vi "MGCC_FntStaMach_main_HTB.vi"() -> ()   [LabVIEW 2016]
doc: "-----------------------------------------------------------------------------------------------------------------------\nCopyright <2019> <The University of Tennessee at Knoxville and the University of Tennessee Research Foundation>\nThis software is released under BSD-3 \nhttps://opensource.org/licenses/BSD-3-Clause \nAdditional license options available at https://utrf.tennessee.edu/industry/sample-agreements/\n-----------------------------------------------------------------------------------------------------------------------\n\n\nMain function for FSM in MGCC. The inputs are flags feedback from other functions and MGLCs. The outputs are the next states and updates in sensoring datas."
panel:
  in  "i_MGCC_StaEst_breakpoint":i32=11
  in  "b_MGCC_StaEst_enable_noise":bool
  in  "b_MGCC_FntStaMach_All_Loop_Stop":bool
  out "Functions":bool[](array[boolean])
  out "Current state":string
  out "Current Time":string
  in  "Manual turn off":bool
  in  "Event manual panel":bool
  out "Bool of state":bool[](array[boolean])
  # "Finte State Machine"
  # "Energy management"
  # "State Esimation"
  # "Model Management"
  # "Data Logging"
  # "Communication"
  # "PV Forecasting"
  # "PQ Balance"
  # "Load Forecasting"
  # "BKS"
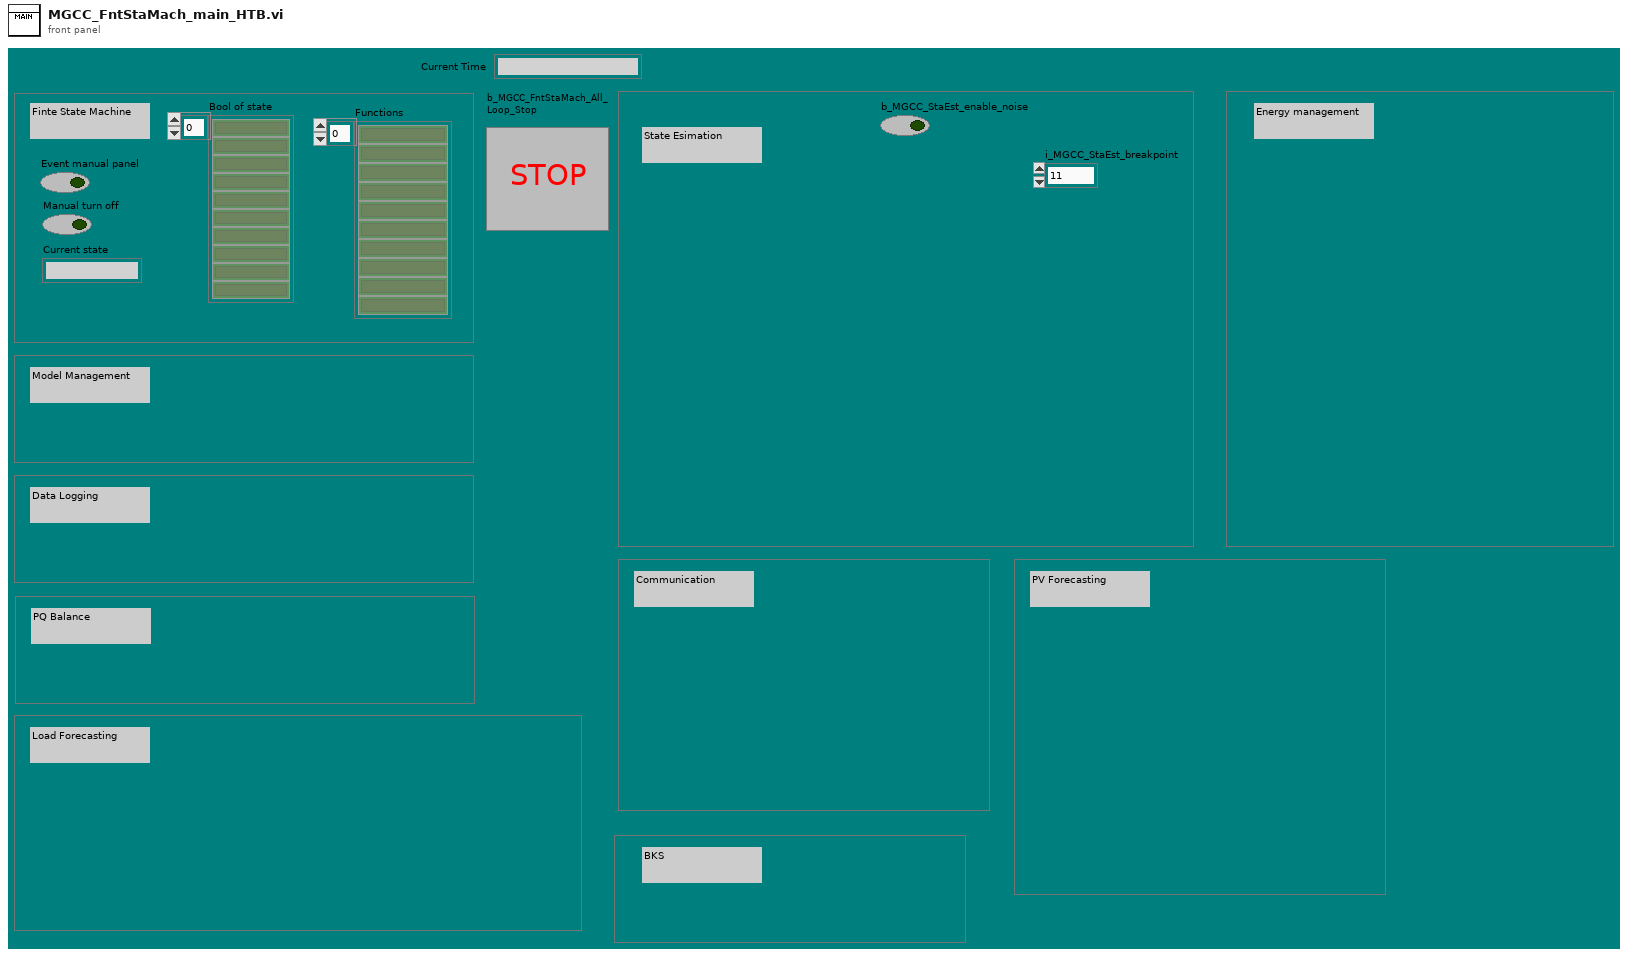
[diagram p1: front panel]
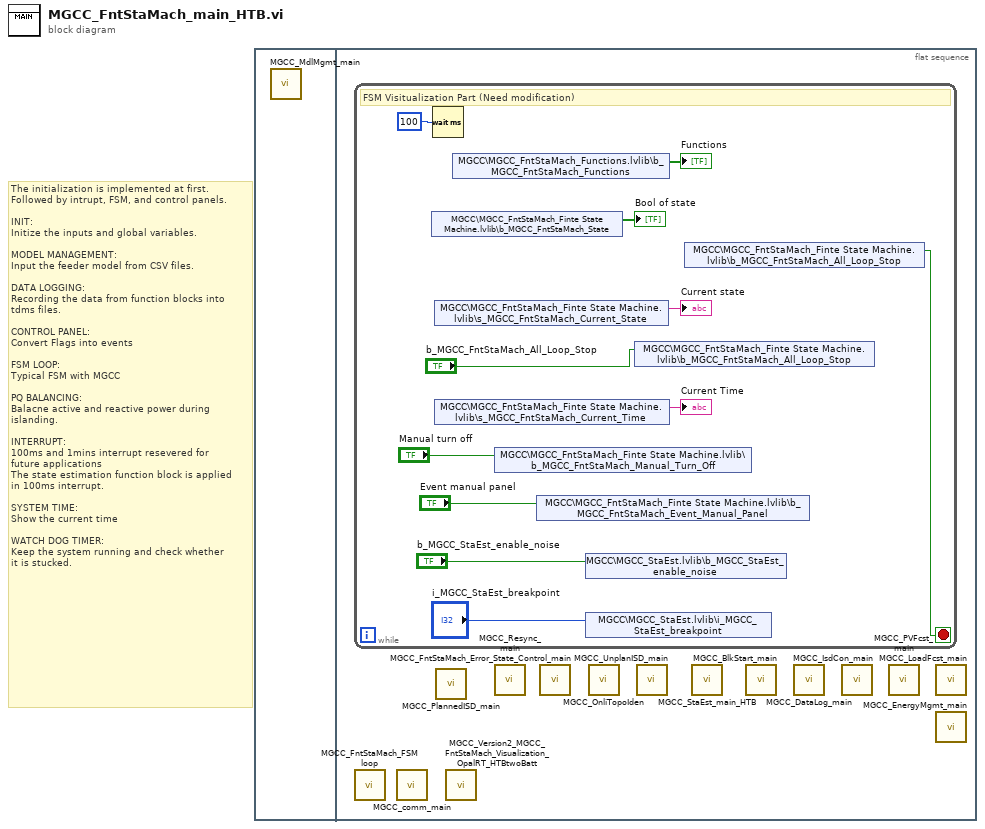
[diagram p0: block diagram]
diagram:
  # "The initialization is implemented at first.\nFollowed by intrupt, FSM, and control panels.\n\nINIT:\nInitize the inputs and global variables.\n\nMODEL MANAGEMENT:\nInput the feeder model from CSV files.\n\nDATA LOGGING:\nRecording the data from function blocks into\ntdms files.\n\nCONTROL PANEL:\nConvert Flags into events\n\nFSM LOOP:\nTypical FSM with MGCC\n\nPQ BALANCING:\nBalacne active and reactive power during \nislanding.\n\nINTERRUPT:\n100ms and 1mins interrupt resevered for \nfuture applications\nThe state estimation function block is applied\nin 100ms interrupt.\n\nSYSTEM TIME:\nShow the current time\n\nWATCH DOG TIMER:\nKeep the system running and check whether\nit is stucked."
  n1 = flat-sequence {
    frame #0 {
      n2 = call "MGCC_MdlMgmt_main.vi"() -> ()  [unwired: 12 in]
    }
    frame #1 {
      n3 = while {
        stop <- w10 stop-if-true
        # "FSM Visitualization Part (Need modification)"
        n4 = shared-variable "MGCC\\MGCC_FntStaMach_Finte State Machine.lvlib\\b_MGCC_FntStaMach_State"() -> (→"Bool of state":bool[])  [unwired: 1 in, 1 out]
        n5 = Wait (ms)(milliseconds to wait=u32 100) -> ()  [unwired: 1 out]
        n6 = shared-variable "MGCC\\MGCC_FntStaMach_Finte State Machine.lvlib\\s_MGCC_FntStaMach_Current_State"() -> (→"Current state":string)  [unwired: 1 in, 1 out]
        n7 = shared-variable "MGCC\\MGCC_FntStaMach_Finte State Machine.lvlib\\s_MGCC_FntStaMach_Current_Time"() -> (→"Current Time":string)  [unwired: 1 in, 1 out]
        n8 = shared-variable "MGCC\\MGCC_FntStaMach_Functions.lvlib\\b_MGCC_FntStaMach_Functions"() -> (→"Functions":bool[])  [unwired: 1 in, 1 out]
        n9 = shared-variable "MGCC\\MGCC_FntStaMach_Finte State Machine.lvlib\\b_MGCC_FntStaMach_Manual_Turn_Off"("Manual turn off") -> ()  [unwired: 1 in, 1 out]
        n10 = shared-variable "MGCC\\MGCC_FntStaMach_Finte State Machine.lvlib\\b_MGCC_FntStaMach_Event_Manual_Panel"("Event manual panel") -> ()  [unwired: 1 in, 1 out]
        n11 = shared-variable "MGCC\\MGCC_StaEst.lvlib\\b_MGCC_StaEst_enable_noise"("b_MGCC_StaEst_enable_noise") -> ()  [unwired: 1 in, 1 out]
        n12 = shared-variable "MGCC\\MGCC_StaEst.lvlib\\i_MGCC_StaEst_breakpoint"("i_MGCC_StaEst_breakpoint") -> ()  [unwired: 1 in, 1 out]
        n13 = shared-variable "MGCC\\MGCC_FntStaMach_Finte State Machine.lvlib\\b_MGCC_FntStaMach_All_Loop_Stop"("b_MGCC_FntStaMach_All_Loop_Stop") -> ()  [unwired: 1 in, 1 out]
        n14 = shared-variable "MGCC\\MGCC_FntStaMach_Finte State Machine.lvlib\\b_MGCC_FntStaMach_All_Loop_Stop"() -> (w10:bool)  [unwired: 1 in, 1 out]
      }
      n15 = call "MGCC_FntStaMach_FSM loop.vi"() -> ()  [unwired: 8 in, 4 out]
      n16 = call "MGCC_comm_main.vi"() -> ()  [unwired: 12 in]
      n17 = call "MGCC_PlannedISD_main.vi"() -> ()  [unwired: 12 in]
      n18 = call "MGCC_Version2_MGCC_FntStaMach_Visualization_OpalRT_HTBtwoBatt.vi"() -> ()  [unwired: 12 in]
      n19 = call "MGCC_Resync_main.vi"() -> ()  [unwired: 12 in]
      n20 = call "MGCC_FntStaMach_Error_State_Control_main.vi"() -> ()  [unwired: 12 in]
      n21 = call "MGCC_OnliTopoIden.vi"() -> ()  [unwired: 12 in]
      n22 = call "MGCC_UnplanISD_main.vi"() -> ()  [unwired: 12 in]
      n23 = call "MGCC_StaEst_main_HTB.vi"() -> ()  [unwired: 12 in]
      n24 = call "MGCC_BlkStart_main.vi"() -> ()  [unwired: 12 in]
      n25 = call "MGCC_DataLog_main.vi"() -> ()  [unwired: 12 in]
      n26 = call "MGCC_IsdCon_main.vi"() -> ()  [unwired: 12 in]
      n27 = call "MGCC_PVFcst_main.vi"() -> ()  [unwired: 12 in]
      n28 = call "MGCC_LoadFcst_main.vi"() -> ()  [unwired: 12 in]
      n29 = call "MGCC_EnergyMgmt_main.vi"() -> ()  [unwired: 12 in]
    }
  }
